vi "q2 binary digit value.vi"(9 "position":dbl, 11 "b":bool) -> (2 "value":dbl)   [LabVIEW 2025]
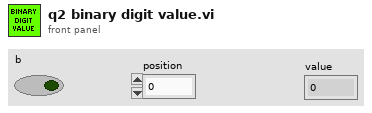
[diagram p1: front panel]
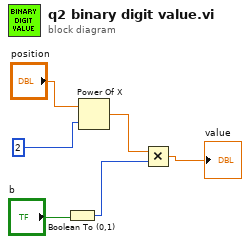
[diagram p0: block diagram]
diagram:
  n1 = Boolean To (0,1)(Boolean="b") -> (0, 1=w4:i16)
  n2 = Power Of X(1:2, 2:"position") -> (0:w5:dbl)
  n3 = Multiply(x=w5, y=w4) -> (x*y=→"value":dbl)
